vi "质控参数保存.vi"(7 "section":string="氨氮质控参数", 8 "error in (no error)":errorcluster caption="错误输入（无错误）", 11 "参数":T1) -> (0 "error out":errorcluster caption="错误输出")   [LabVIEW 2016, in "质控单元.lvlib"]
uses:
  <vilib>/Utility/config.llb/Write Key (Double).vi
  <vilib>/Utility/config.llb/NI_LVConfig.lvlib
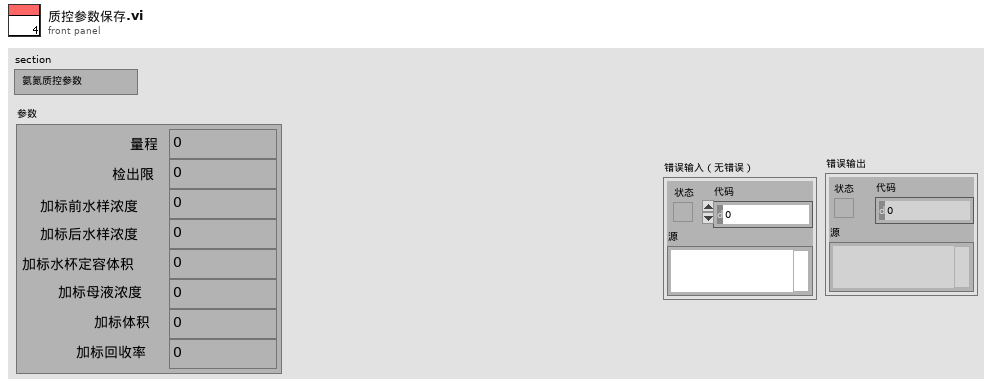
[diagram p1: front panel]
types:
  T1 = cluster{"量程":dbl, "检出限":dbl, "加标前水样浓度":dbl, "加标后水样浓度":dbl, "加标水杯定容体积":dbl, "加标母液浓度":dbl, "加标体积":dbl, "加标回收率":dbl}
  T2 = typedef "NI_LVConfig.lvlib/Config Data RefNum.ctl" = refnum<k1>
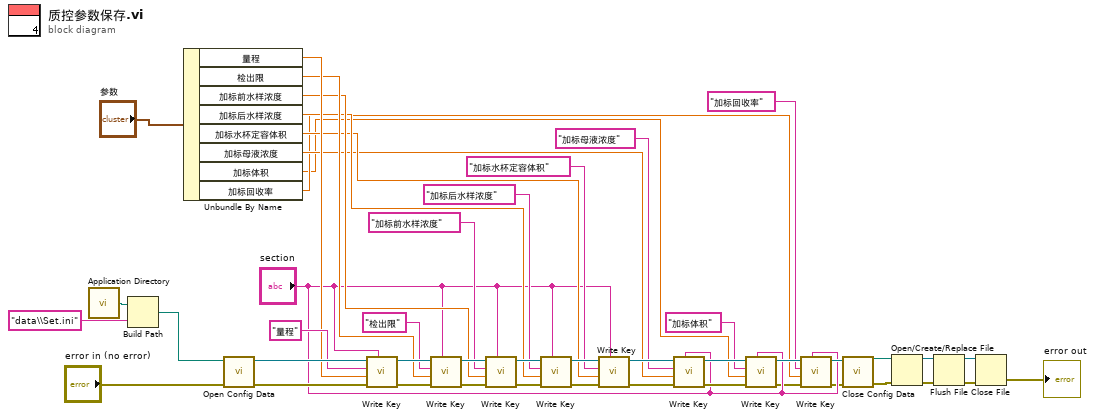
[diagram p0: block diagram]
diagram:
  n1 = call <vilib>:"Application Directory.vi"() -> ("Application Directory"=w45:path)
  n2 = Build Path(base path=w45, name or relative path="data\\Set.ini" ("名称或相对路径")) -> (appended path=w43:path)
  n3 = Unbundle By Name("参数") -> ("量程"=w24:dbl, "检出限"=w23:dbl, "加标前水样浓度"=w22:dbl, "加标后水样浓度"=w21:dbl, "加标水杯定容体积"=w20:dbl, "加标母液浓度"=w19:dbl, "加标体积"=w8:dbl, "加标回收率"=w9:dbl)
  n4 = call <vilib>:"Open Config Data.vi"("error in (no error)"="error in (no error)", "configuration file path"=w43) -> ("error out"=w46:errorcluster, "refnum"=w47:T2)  [unwired: 7 in, 1 out]
  n5 = call-poly <vilib>:"Write Key.vi"("section"="section", "error in (no error)"=w46, "value"=w24, "key"="量程", "refnum"=w47) -> ("error out"=w40:errorcluster, "refnum out"=w41:T2)  [unwired: 4 in, 1 out]
  n6 = call-poly <vilib>:"Write Key.vi"("section"="section", "error in (no error)"=w40, "value"=w23, "key"="检出限", "refnum"=w41) -> ("error out"=w38:errorcluster, "refnum out"=w39:T2)  [unwired: 4 in, 1 out]
  n7 = call-poly <vilib>:"Write Key.vi"("section"="section", "error in (no error)"=w38, "value"=w22, "key"="加标前水样浓度", "refnum"=w39) -> ("error out"=w32:errorcluster, "refnum out"=w33:T2)  [unwired: 4 in, 1 out]
  n8 = call-poly <vilib>:"Write Key.vi"("section"="section", "error in (no error)"=w32, "value"=w21, "key"="加标后水样浓度", "refnum"=w33) -> ("error out"=w35:errorcluster, "refnum out"=w34:T2)  [unwired: 4 in, 1 out]
  n9 = call-poly <vilib>:"Write Key.vi"("section"="section", "error in (no error)"=w35, "value"=w20, "key"="加标水杯定容体积", "refnum"=w34) -> ("error out"=w37:errorcluster, "refnum out"=w36:T2)  [unwired: 4 in, 1 out]
  n10 = call-poly <vilib>:"Write Key.vi"("section"="section", "error in (no error)"=w37, "value"=w19, "key"="加标母液浓度", "refnum"=w36) -> ("error out"=w18:errorcluster, "refnum out"=w17:T2)  [unwired: 4 in, 1 out]
  n11 = call-poly <vilib>:"Write Key.vi"("section"="section", "error in (no error)"=w18, "value"=w8, "key"="加标体积", "refnum"=w17) -> ("error out"=w11:errorcluster, "refnum out"=w16:T2)  [unwired: 4 in, 1 out]
  n12 = call-poly <vilib>:"Write Key.vi"("section"="section", "error in (no error)"=w11, "value"=w9, "key"="加标回收率", "refnum"=w16) -> ("error out"=w10:errorcluster, "refnum out"=w15:T2)  [unwired: 4 in, 1 out]
  n13 = call <vilib>:"Close Config Data.vi"("error in (no error)"=w10, "refnum"=w15) -> ("error out"=w3:errorcluster, "file path"=w2:path)  [unwired: 8 in]
  n14 = Open/Create/Replace File(file path (use dialog)=w2, error in=w3) -> (refnum out=w5:refnum<file>, error out=w4:errorcluster)  [unwired: 4 in, 1 out]
  n15 = Flush File(refnum=w5, error in=w4) -> (refnum out=w6:refnum<file>, error out=w7:errorcluster)
  n16 = Close File(refnum=w6, error in=w7) -> (error out=→"error out":errorcluster)  [unwired: 1 out]
